vi "X axial.vi"(8 "曲线名称":string[](array[string]), 9 "曲线数量":u32, 10 "频率配置":i32, 11 "当前混响频谱图":refnum<vi>) -> (2 "所有X坐标":dbl[](array[numeric]))   [LabVIEW 2020]
panel:
  out "大小":i32
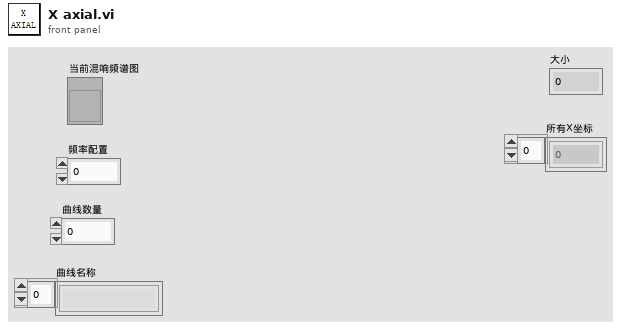
[diagram p1: front panel]
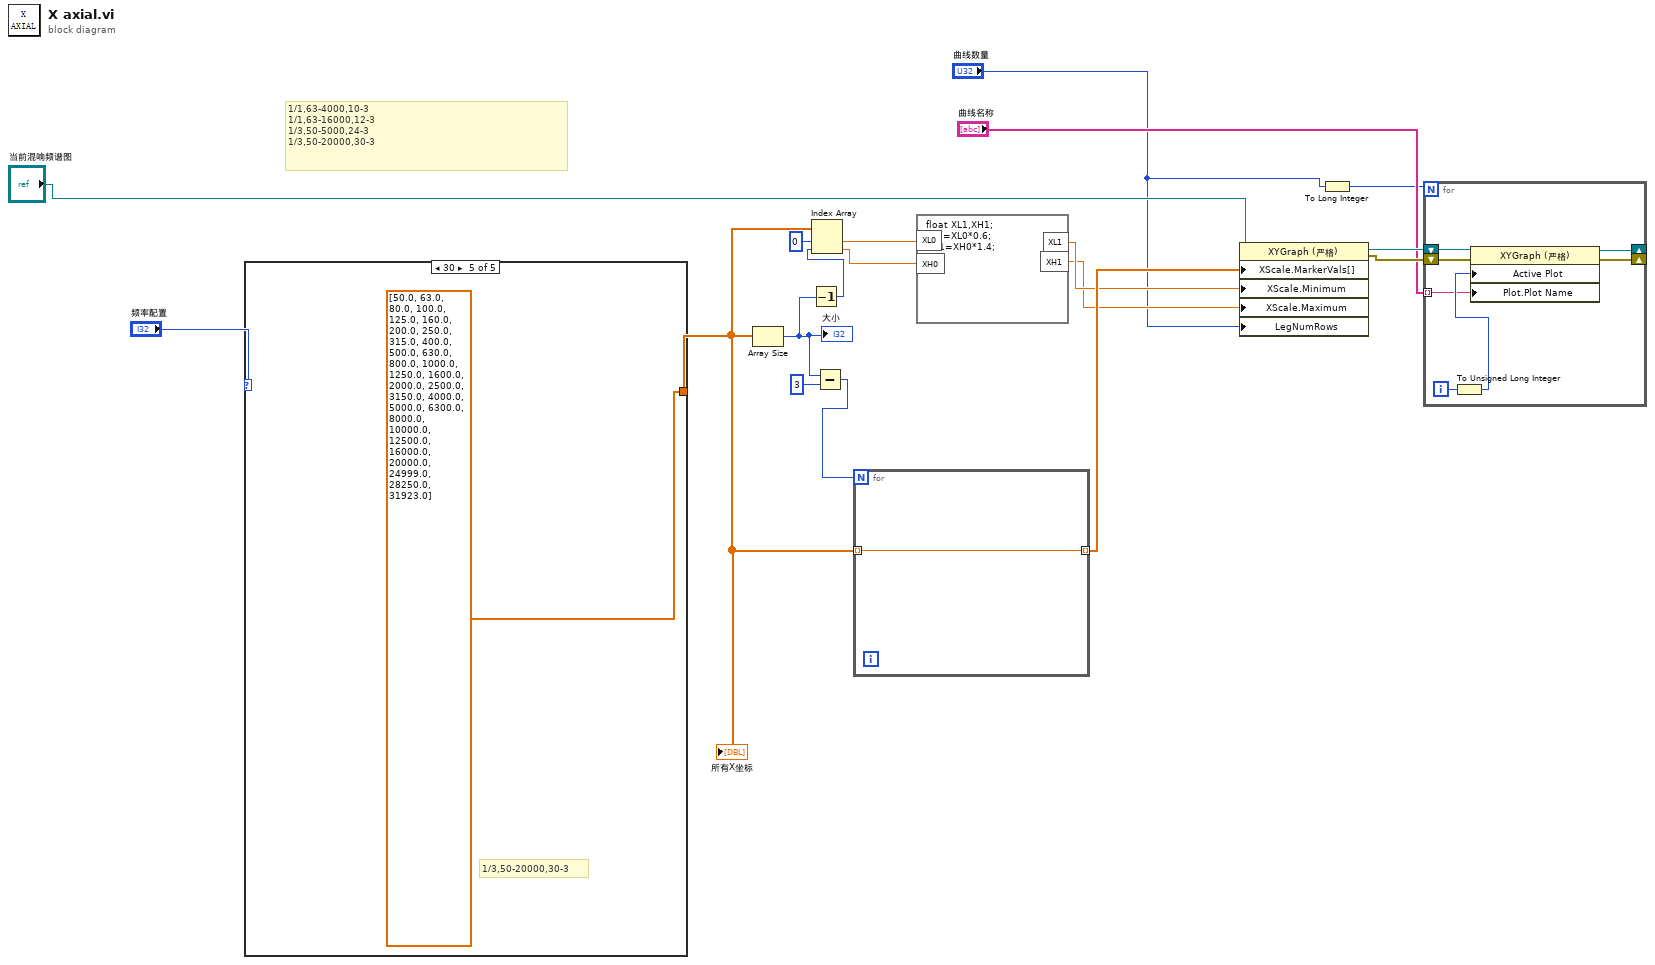
[diagram p0: block diagram]
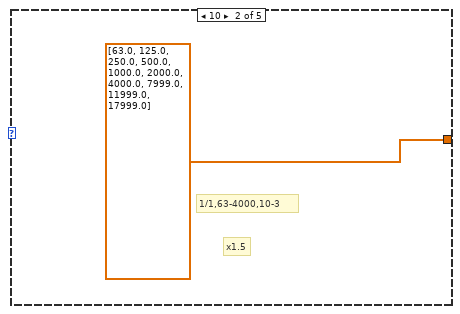
[diagram p3: hidden frame]
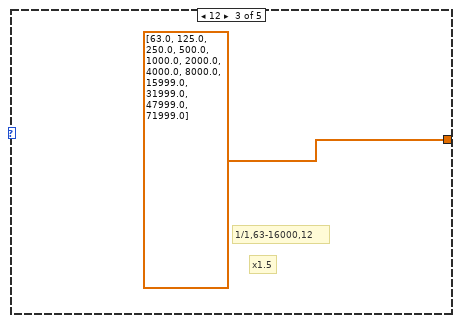
[diagram p4: hidden frame]
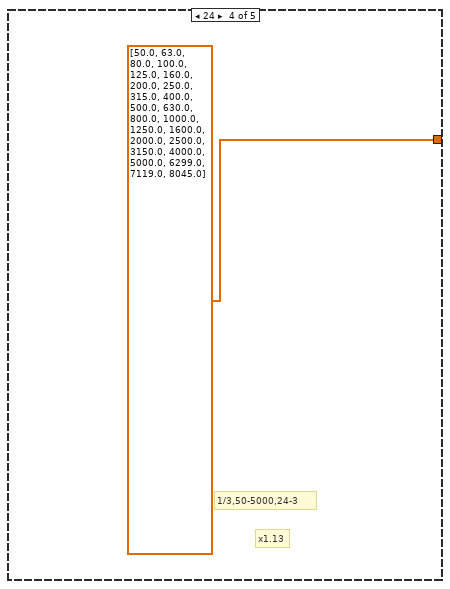
[diagram p5: hidden frame]
diagram:
  # "1/1,63-4000,10-3\n1/1,63-16000,12-3\n1/3,50-5000,24-3\n1/3,50-20000,30-3"
  n1 = case shown="30" "频率配置" {
    tunnel: [_ dbl[] [63.0, 125.0, 250.0, 500.0, 1000.0, 2000.0, 4000.0, 7999.0, 11999.0, 17999.0] dbl[] [63.0, 125.0, 250.0, 500.0, 1000.0, 2000.0, 4000.0, 8000.0, 15999.0, 31999.0, 47999.0, 71999.0] dbl[] [50.0, 63.0, 80.0, 100.0, 125.0, 160.0, 200.0, 250.0, 315.0, 400.0, 500.0, 630.0, 800.0, 1000.0, 1250.0, 1600.0, 2000.0, 2500.0, 3150.0, 4000.0, 5000.0, 6299.0, 7119.0, 8045.0] dbl[] [50.0, 63.0, 80.0, 100.0, 125.0, 160.0, 200.0, 250.0, 315.0, 400.0, 500.0, 630.0, 800.0, 1000.0, 1250.0, 1600.0, 2000.0, 2500.0, 3150.0, 4000.0, 5000.0, 6300.0, 8000.0, 10000.0, 12500.0, 16000.0, 20000.0, 24999.0, 28250.0, 31923.0]] -> w14
    frame 0, Default {
      # "1/1,63-4000,10"
    }
    frame 10 {
      # "x1.5"
      # "1/1,63-4000,10-3"
    }
    frame 12 {
      # "x1.5"
      # "1/1,63-16000,12"
    }
    frame 24 {
      # "x1.13"
      # "1/3,50-5000,24-3"
    }
    frame 30 {
      # "1/3,50-20000,30-3"
    }
  }
  "所有X坐标" <- w14
  n2 = Array Size(array=w14) -> (size(s)=w8:i32)
  "大小" <- w8
  n3 = Decrement(x=w8) -> (x-1=w7:i32)
  n4 = Index Array(array=w14, index #1=0 ("索引"), index #2=w7) -> (element #1=w12:dbl, element #2=w11:dbl)
  n5 = Subtract(x=w8, y=3) -> (x-y=w16:i32)
  n6 = for {
    N: w16 -> [_]
    tunnel: w14 -> [w23] mode=indexing
    tunnel: [w23] -> w15 mode=indexing
  }
  n7 = formula code="float XL1,XH1;\nXL1=XL0*0.6;\nXH1=XH0*1.4;"("XL0"=w12, "XH0"=w11) -> ("XL1"=w10:dbl, "XH1"=w9:dbl)
  n8 = property class="XYGraph (严格)"(reference="当前混响频谱图", "XScale.MarkerVals[]"=w15, "XScale.Minimum"=w10, "XScale.Maximum"=w9, "LegNumRows"="曲线数量") -> (reference out=w5:refnum<vi>, error out=w4:errorcluster)  [unwired: 1 in]
  n9 = To Long Integer(number="曲线数量") -> (32bit integer=w1:i32)
  n10 = for {
    N: w1 -> [_]
    shift-right: [w28] -> _
    shift-left: w5 -> [w30]
    shift-right: [w27] -> _
    shift-left: w4 -> [w29]
    tunnel: "曲线名称" -> [w24] mode=indexing
    i -> [w26]
    n11 = To Unsigned Long Integer(number=w26) -> (unsigned 32bit integer=w25:u32)
    n12 = property class="XYGraph (严格)"(reference=w30, error in=w29, "Active Plot"=w25, "Plot.Plot Name"=w24) -> (reference out=w28:refnum<vi>, error out=w27:errorcluster)
  }
